vi "ViewFIFOSet.vi"(1 "Path":path, 2 "Enum":T4(ring)) -> (0 "FIFO Settings (Array)":T2[](array[typedef]) {"CFD"."CFD Holdoff (ns)" min=5 max=20 format="%.2f"; "CFD"."CFD ZC Level (mV)" min=-96 max=96 format="%.2f"; "CFD"."CFD Limit High (mV)" min=4 max=80 format="%.2f"; "CFD"."CFD Limit Low (mV)" min=-500 max=80 format="%.2f"; "TAC"."TAC Limit High (%)" min=0 max=100 format="%.2f"; "TAC"."TAC Limit Low (%)" min=0 max=100 format="%.2f"; "TAC"."TAC Offset (%)" min=0 max=100 format="%.2f"; "TAC"."TAC Gain" min=1 max=15 step=1; "TAC"."TAC Range (ns)" min=50 max=2000 format="%.2f"; "SYNC"."SYNC Threshold (mV)" min=-500 max=-19 format="%.2f"; "SYNC"."SYNC Holdoff (ns)" min=4 max=16 format="%.2f"; "SYNC"."SYNC Freq Divider" min=1 max=16 step=1; "SYNC"."SYNC ZC Level (mV)" min=-96 max=96 format="%.2f"; "ADC"."Macro Time Clock" items=["Internal (50ns)", "Sync-Trigger", "1/2 Sync-Trigger"]; "ADC"."Module" items=["SPC 630", "SPC 830", "SPC 13x", "HydraHarp"]; "ADC"."Count Increment" min=1 max=255 step=1; "ADC"."Dither Range" min=0 max=256 step=32; "Measurement"."Ext Latch Delay" min=0 max=255 step=1; "Measurement"."Stop Count" format="%.2f"; "Measurement"."Stop Condition:" items=["None", "Photon Count", "Time (s)"]; "Measurement"."External Trigger Condition" max=2 step=1; "Measurement"."No of Channels" max=14; "Measurement"."Binning (ms)" min=1e-07 max=100000 format="%.3f"})   [LabVIEW 2009]
uses:
  FIFOSettings_BH.ctt
  ImageSettings.ctt
  <vilib>/Utility/xml.llb/Read From XML File(string).vi
panel:
  in  "output cluster":T3 {"Image Settings"."2nd Axis" items=["x", "y", "z"]; "Image Settings"."1st Axis" items=["x", "y", "z"]; "Image Settings"."Time Resolution\n(ms/pixel)" format="%.2f"; "Image Settings"."Image Resolution (nm/pixel)"."z" format="%.2f"; "Image Settings"."Image Resolution (nm/pixel)"."y" format="%.2f"; "Image Settings"."Image Resolution (nm/pixel)"."x" format="%.2f"; "Image Settings"."Image Size (µm)"."z" format="%.2f"; "Image Settings"."Image Size (µm)"."y" format="%.2f"; "Image Settings"."Image Size (µm)"."x" format="%.2f"; "Image Settings"."End Position (µm)"."z" format="%.2f"; "Image Settings"."End Position (µm)"."y" format="%.2f"; "Image Settings"."End Position (µm)"."x" format="%.2f"; "Image Settings"."Start Position (µm)"."z" format="%.2f"; "Image Settings"."Start Position (µm)"."y" format="%.2f"; "Image Settings"."Start Position (µm)"."x" format="%.2f"; "FIFO Settings"."CFD"."CFD Holdoff (ns)" min=5 max=20 format="%.2f"; "FIFO Settings"."CFD"."CFD ZC Level (mV)" min=-96 max=96 format="%.2f"; "FIFO Settings"."CFD"."CFD Limit High (mV)" min=4 max=80 format="%.2f"; "FIFO Settings"."CFD"."CFD Limit Low (mV)" min=-500 max=80 format="%.2f"; "FIFO Settings"."TAC"."TAC Limit High (%)" min=0 max=100 format="%.2f"; "FIFO Settings"."TAC"."TAC Limit Low (%)" min=0 max=100 format="%.2f"; "FIFO Settings"."TAC"."TAC Offset (%)" min=0 max=100 format="%.2f"; "FIFO Settings"."TAC"."TAC Gain" min=1 max=15 step=1; "FIFO Settings"."TAC"."TAC Range (ns)" min=50 max=2000 format="%.2f"; "FIFO Settings"."SYNC"."SYNC Threshold (mV)" min=-500 max=-19 format="%.2f"; "FIFO Settings"."SYNC"."SYNC Holdoff (ns)" min=4 max=16 format="%.2f"; "FIFO Settings"."SYNC"."SYNC Freq Divider" min=1 max=16 step=1; "FIFO Settings"."SYNC"."SYNC ZC Level (mV)" min=-96 max=96 format="%.2f"; "FIFO Settings"."ADC"."Macro Time Clock" items=["Internal (50ns)", "Sync-Trigger", "1/2 Sync-Trigger"]; "FIFO Settings"."ADC"."Module" items=["SPC 630", "SPC 830", "SPC 13x", "HydraHarp"]; "FIFO Settings"."ADC"."Count Increment" min=1 max=255 step=1; "FIFO Settings"."ADC"."Dither Range" min=0 max=256 step=32; "FIFO Settings"."Measurement"."Ext Latch Delay" min=0 max=255 step=1; "FIFO Settings"."Measurement"."Stop Count" format="%.2f"; "FIFO Settings"."Measurement"."Stop Condition:" items=["None", "Photon Count", "Time (s)"]; "FIFO Settings"."Measurement"."External Trigger Condition" max=2 step=1; "FIFO Settings"."Measurement"."No of Channels" max=14; "FIFO Settings"."Measurement"."Binning (ms)" min=1e-07 max=100000 format="%.3f"}
  in  "OK Button":bool
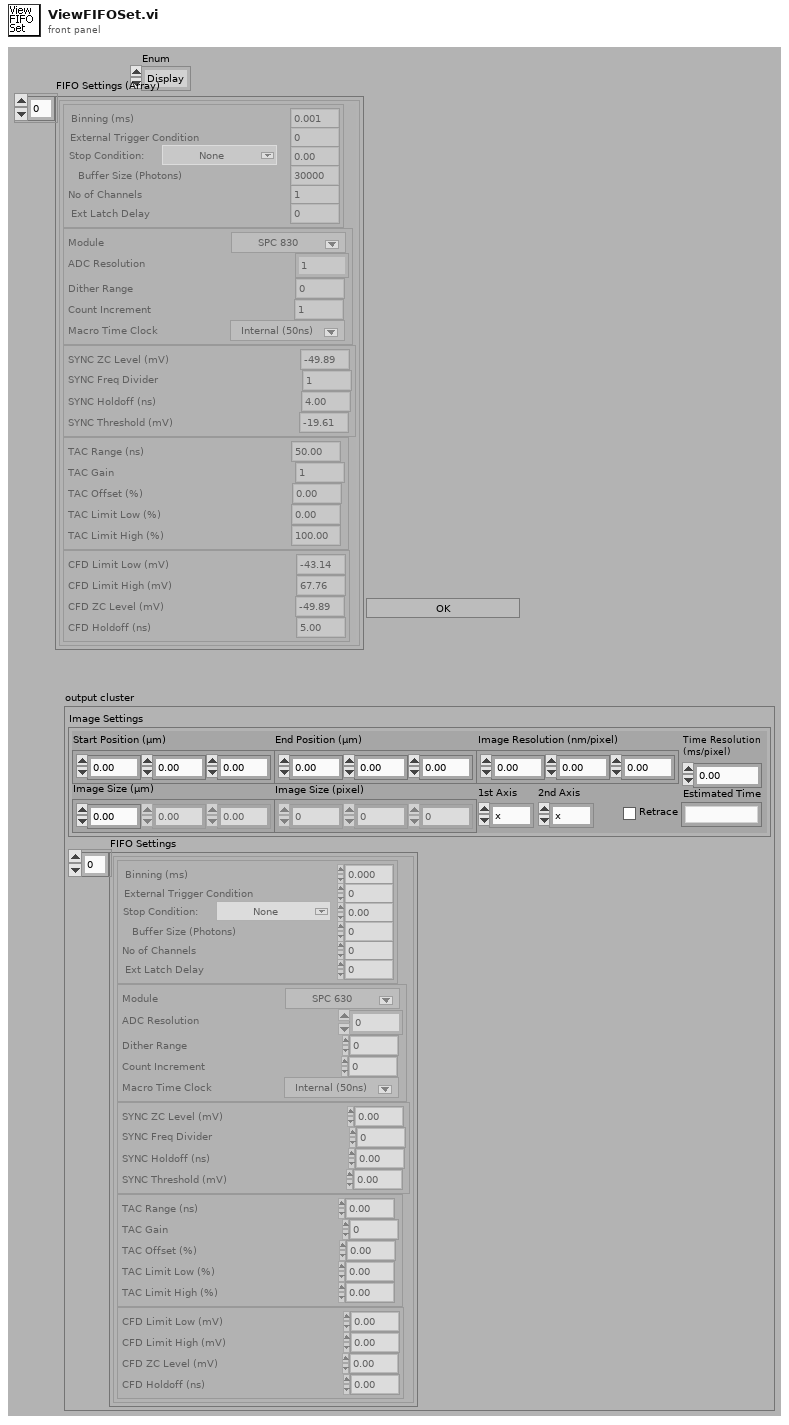
[diagram p1: front panel]
types:
  T1 = typedef "ImageSettings.ctt" = cluster{"Start Position (µm)":cluster{"x":dbl, "y":dbl, "z":dbl}, "End Position (µm)":cluster{"x":dbl, "y":dbl, "z":dbl}, "Image Resolution (nm/pixel)":cluster{"x":dbl, "y":dbl, "z":dbl}, "Image Size (µm)":cluster{"x":dbl, "y":dbl, "z":dbl}, "Image Size (pixel)":cluster{"x":u32, "y":u32, "z":u32}, "Time Resolution\n(ms/pixel)":dbl, "1st Axis":u16, "2nd Axis":u16, "Retrace":bool, "Estimated Time":string}
  T2 = typedef "FIFOSettings_BH.ctt" = cluster{"Measurement":cluster{"Binning (ms)":sgl, "External Trigger Condition":u16, "Stop Condition:":u16, "Stop Count":dbl, "Buffer Size (Photons)":u16, "No of Channels":u16, "Ext Latch Delay":i16}, "ADC":cluster{"Module":u16, "ADC Resolution":i32, "Dither Range":i16, "Count Increment":i16, "Macro Time Clock":i16}, "SYNC":cluster{"SYNC ZC Level (mV)":sgl, "SYNC Freq Divider":i16, "SYNC Holdoff (ns)":sgl, "SYNC Threshold (mV)":sgl}, "TAC":cluster{"TAC Range (ns)":sgl, "TAC Gain":i16, "TAC Offset (%)":sgl, "TAC Limit Low (%)":sgl, "TAC Limit High (%)":sgl}, "CFD":cluster{"CFD Limit Low (mV)":sgl, "CFD Limit High (mV)":sgl, "CFD ZC Level (mV)":sgl, "CFD Holdoff (ns)":sgl}}
  T3 = cluster{"Image Settings":T1, "FIFO Settings":T2[]}
  T4 = enum16{"Display", "change", "Get", "Set", "Set Ken"}
  T5 = cluster{"Image Settings":T1, cluster{"Measurement":cluster{"Binning (ms)":sgl, "External Trigger Condition":u16, "Stop Condition:":u16, "Stop Count":dbl, "Buffer Size (Photons)":u16, "No of Channels":u16, "Ext Latch Delay":i16}, "ADC":cluster{"Module":u16, "ADC Resolution":i32, "Dither Range":i16, "Count Increment":i16, "Macro Time Clock":i16}, "SYNC":cluster{"SYNC ZC Level (mV)":sgl, "SYNC Freq Divider":i16, "SYNC Holdoff (ns)":sgl, "SYNC Threshold (mV)":sgl}, "TAC":cluster{"TAC Range (ns)":sgl, "TAC Gain":i16, "TAC Offset (%)":sgl, "TAC Limit Low (%)":sgl, "TAC Limit High (%)":sgl}, "CFD":cluster{"CFD Limit Low (mV)":sgl, "CFD Limit High (mV)":sgl, "CFD ZC Level (mV)":sgl, "CFD Holdoff (ns)":sgl}}[]}
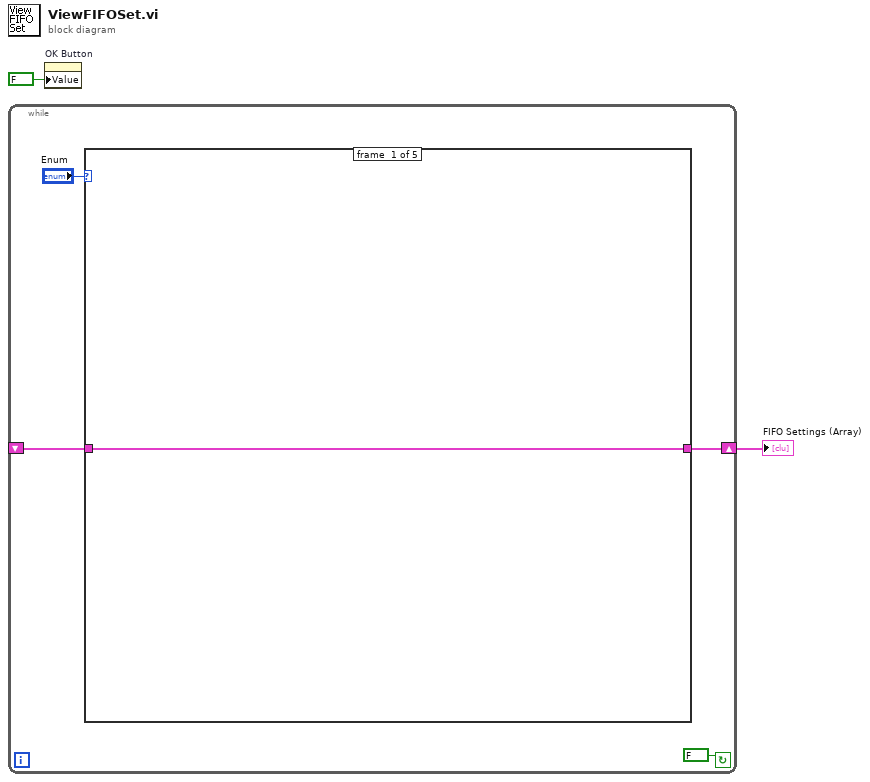
[diagram p0: block diagram]
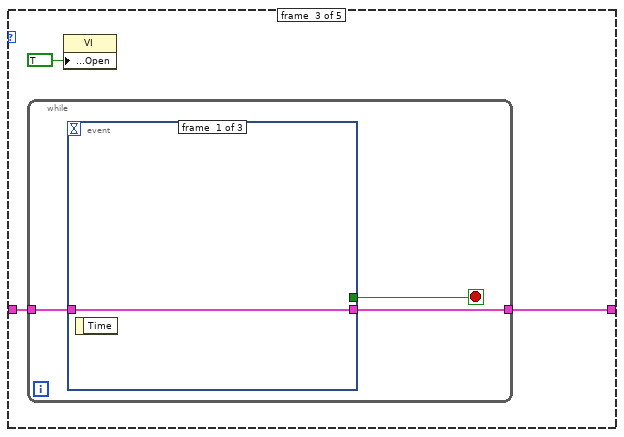
[diagram p3: hidden frame]
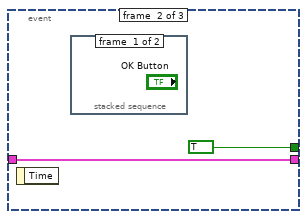
[diagram p4: hidden frame]
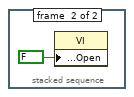
[diagram p5: hidden frame]
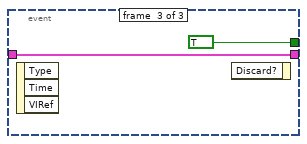
[diagram p6: hidden frame]
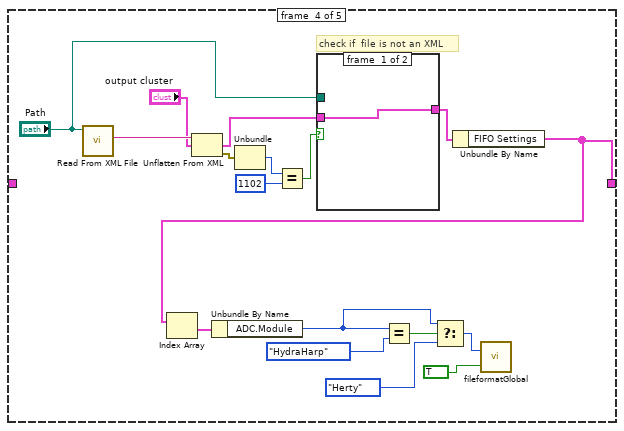
[diagram p7: hidden frame]
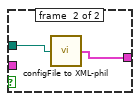
[diagram p8: hidden frame]
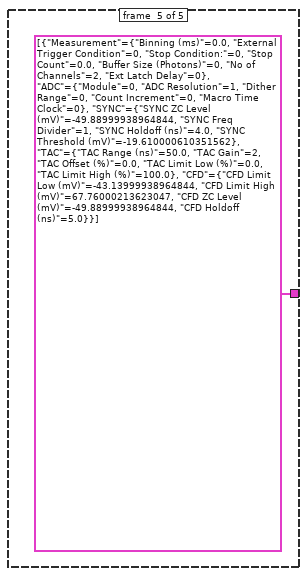
[diagram p9: hidden frame]
diagram:
  n1 = while {
    shift-right: [w4] -> w1
    shift-left: _ -> [w5]
    stop <- FALSE continue-if-true
    n2 = case shown="\"Set\"" "Enum" {
      tunnel: w5 -> [w7 w8 w10 _ _]
      tunnel: [w7 w8 w9 w35 T2[] [{"Measurement"={"Binning (ms)"=0.0, "External Trigger Condition"=0, "Stop Condition:"=0, "Stop Count"=0.0, "Buffer Size (Photons)"=0, "No of Channels"=2, "Ext Latch Delay"=0}, "ADC"={"Module"=0, "ADC Resolution"=1, "Dither Range"=0, "Count Increment"=0, "Macro Time Clock"=0}, "SYNC"={"SYNC ZC Level (mV)"=-49.89, "SYNC Freq Divider"=1, "SYNC Holdoff (ns)"=4.0, "SYNC Threshold (mV)"=-19.61}, "TAC"={"TAC Range (ns)"=50.0, "TAC Gain"=2, "TAC Offset (%)"=0.0, "TAC Limit Low (%)"=0.0, "TAC Limit High (%)"=100.0}, "CFD"={"CFD Limit Low (mV)"=-43.14, "CFD Limit High (mV)"=67.76, "CFD ZC Level (mV)"=-49.89, "CFD Holdoff (ns)"=5.0}}]] -> w4
      frame #0 {
      }
      frame #1 {
      }
      frame #2 {
        n3 = while {
          tunnel: w10 -> [w13]
          tunnel: [w12] -> w9
          stop <- w14 stop-if-true
          n4 = event shown="[2] Panel Close?" {
            selector: _ -> [_ _ _]
            dyn-events: _ -> [_ _ _]
            timeout: _ -> [_ _ _]
            tunnel: [_ TRUE TRUE] -> w14
            tunnel: w13 -> [w15 w16 w19]
            tunnel: [w15 w16 w19] -> w12
            event #0 {
              n5 = event-data() -> ()  [unwired: 1 in, 1 out]
            }
            event #1 {
              n6 = event-data() -> ()  [unwired: 1 in, 1 out]
              n7 = stacked-sequence {
                frame #0 {
                }
                frame #1 {
                  n8 = property class="VI"("Front Panel Window:Open"=FALSE) -> ()  [unwired: 2 in, 2 out]
                }
              }
            }
            event #2 {
              n9 = event-data() -> ()  [unwired: 1 in, 3 out]
              n10 = event-data() -> ()  [unwired: 2 in, 1 out]
            }
          }
        }
        n11 = property class="VI"("Front Panel Window:Open"=TRUE) -> ()  [unwired: 2 in, 2 out]
      }
      frame #3 {
        # "check if  file is not an XML"
        n12 = call-poly <vilib>:"Read From XML File.vi"("XML File Path"="Path") -> ("XML Elements"=w37:string)  [unwired: 8 in, 2 out]
        n13 = Unflatten From XML(xml string=w37, type="output cluster") -> (value=w22:T3, error out=w27:errorcluster)  [unwired: 1 in]
        n14 = Unbundle(w27) -> ("code"=w26:i32)  [unwired: 2 out]
        n15 = Equal?(x=w26, y=1102) -> (x = y?=w24:bool)
        n16 = case shown="True" w24 {
          tunnel: [w38 w39] -> w23
          tunnel: w22 -> [w38 _]
          tunnel: "Path" -> [_ w40]
          frame #0 {
          }
          frame #1 {
            n17 = call "configFile to XML-phil.vi"("configuration file path"=w40) -> ("output cluster"=w39:T5)
          }
        }
        n18 = Unbundle By Name(w23) -> ("FIFO Settings"=w35:T2[])
        n19 = Index Array(array=w35) -> (element=w34:T2)  [unwired: 1 in]
        n20 = Unbundle By Name(w34) -> ("ADC.Module"=w30:u16)
        n21 = Equal?(x=w30, y=enum16{"Herty", "Ken", "SPC130", "HydraHarp"}."HydraHarp" ("Fileformat")) -> (x = y?=w31:bool)
        n22 = Select(t=w30, s=w31, f=enum16{"Herty", "Ken", "SPC130", "HydraHarp"}."Herty" ("Fileformat")) -> (s? t:f=w28:u16)
        n23 = call "fileformatGlobal.vi"("changed"=TRUE, "Fileformat"=w28) -> ()  [unwired: 1 out]
      }
      frame #4 {
      }
    }
  }
  "FIFO Settings (Array)" <- w1
  n24 = property on="OK Button" class="Boolean"("Value"=FALSE ("Visible")) -> ()  [unwired: 2 in, 2 out]
